vi "Update Stim Pattern.vi"(0 "Stim Pattern In":T1[][](array[typedef])=[[enum."Full", enum."Half", enum."Off", enum."Off", enum."Off", enum."Off", enum."Half"], [enum."Full", enum."Off", enum."Off", enum."Off", enum."Off", enum."Half", enum."Half"], [enum."Half", enum."Full", enum."Off", enum."Full", enum."Off", enum."Off", enum."Full"], [enum."Half", enum."Off", enum."Off", enum."Half", enum."Full", enum."Full", enum."Full"], [enum."Off", enum."Full", enum."Half", enum."Half", enum."Off", enum."Off", enum."Off"]]) -> (1 "Stim Pattern Out":T1[][](array[typedef])=[[enum."Full", enum."Half", enum."Off", enum."Off", enum."Off", enum."Off", enum."Half"], [enum."Full", enum."Off", enum."Off", enum."Off", enum."Off", enum."Half", enum."Half"], [enum."Half", enum."Full", enum."Off", enum."Full", enum."Off", enum."Off", enum."Full"], [enum."Half", enum."Off", enum."Off", enum."Half", enum."Full", enum."Full", enum."Full"], [enum."Off", enum."Full", enum."Half", enum."Half", enum."Off", enum."Off", enum."Off"]], 2 "Pretty Colors Out":u32[][](array[colorbox]))   [LabVIEW 2019]
uses:
  Gait Phase Names.ctl
  Stim off-half-ful.ctl
  Muscle Group Labels.ctl
panel:
  out "Pretty Colors Display":T4={"Muscle Group Labels"=["Muscle Groups", "Gluteals", "Hamstrings", "Quadriceps", "Tibialis Anterior", "Triceps Surae"], "Cluster"={"Gait Phases  "=["LR", "MSt", "TSt", "PSw", "ISw", "MSw", "TSw"], "Pretty Colors"=[]}}
  in  "Stim Pattern Control":T5={"_"={"Array 3"=["Muscle Groups"], "Array 2"=["Gluteals", "Hamstrings", "Quadriceps", "Tibialis Anterior", "Triceps Surae"]}, "Stimulation Pattern"={"Gait Phases  "=["LR", "MSt", "TSt", "PSw", "ISw", "MSw", "TSw"], "Values"=[[enum."Full", enum."Half", enum."Off", enum."Off", enum."Off", enum."Off", enum."Half"], [enum."Full", enum."Off", enum."Off", enum."Off", enum."Off", enum."Half", enum."Half"], [enum."Half", enum."Full", enum."Off", enum."Full", enum."Off", enum."Off", enum."Full"], [enum."Half", enum."Off", enum."Off", enum."Half", enum."Full", enum."Full", enum."Full"], [enum."Off", enum."Full", enum."Half", enum."Half", enum."Off", enum."Off", enum."Off"]]}}
  in  "F'n Done":bool
  # "Edit Here"
  # "Pretty Colors"
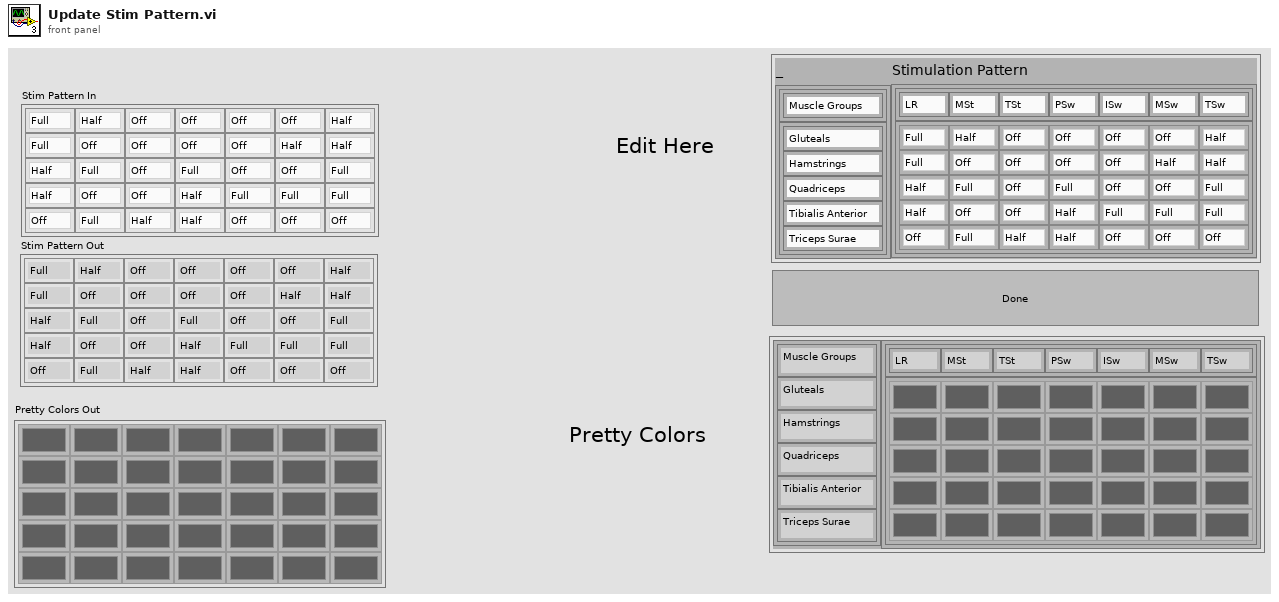
[diagram p1: front panel]
types:
  T1 = typedef "Stim off-half-ful.ctl" = enum16{"Off", "Half", "Full"}
  T2 = typedef "Muscle Group Labels.ctl" = string[]
  T3 = typedef "Gait Phase Names.ctl" = string[]
  T4 = cluster{"Muscle Group Labels":T2, "Cluster":cluster{"Gait Phases  ":T3, "Pretty Colors":u32[][]}}
  T5 = cluster{"_":cluster{"Array 3":string[], "Array 2":string[]}, "Stimulation Pattern":cluster{"Gait Phases  ":T3, "Values":T1[][]}}
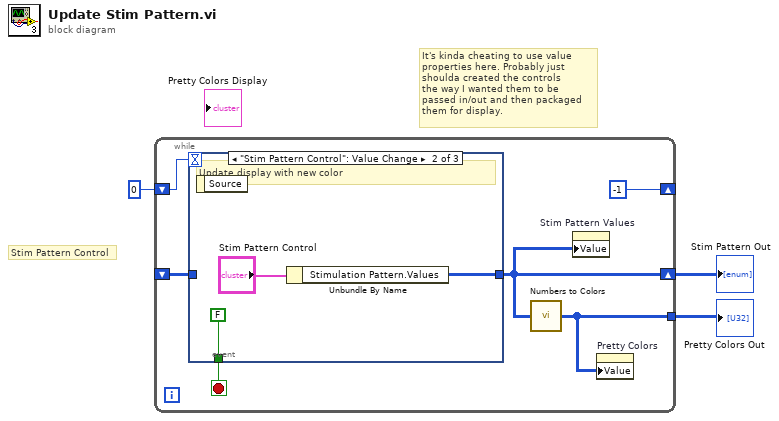
[diagram p0: block diagram]
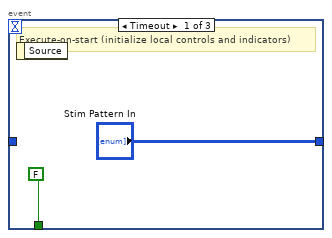
[diagram p2: hidden frame]
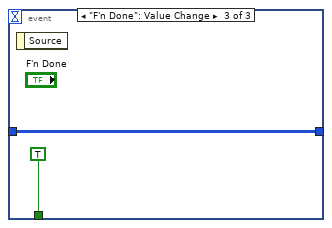
[diagram p3: hidden frame]
diagram:
  # "It's kinda cheating to use value\nproperties here. Probably just\nshoulda created the controls\nthe way I wanted them to be\npassed in/out and then packaged\nthem for display."
  # "Stim Pattern Control"
  n1 = while {
    shift-right: [-1] -> _
    shift-left: 0 -> [w8]
    shift-right: [w6] -> w2
    shift-left: _ -> [w5]
    tunnel: [w4] -> w1
    stop <- w9 stop-if-true
    n2 = event shown="[1] \"Stim Pattern Control\": Value Change" {
      selector: _ -> [_ _ _]
      dyn-events: _ -> [_ _ _]
      timeout: w8 -> [_ _ _]
      tunnel: [FALSE FALSE TRUE] -> w9
      tunnel: ["Stim Pattern In" w12 w15] -> w6
      tunnel: w5 -> [_ _ w15]
      event Timeout {
        # "Execute-on-start (initialize local controls and indicators)"
        n3 = event-data() -> ()  [unwired: 1 in, 1 out]
      }
      event "Stim Pattern Control": Value Change {
        # "Update display with new color"
        n4 = event-data() -> ()  [unwired: 1 in, 1 out]
        n5 = Unbundle By Name("Stim Pattern Control") -> ("Stimulation Pattern.Values"=w12:T1[][])
      }
      event "F'n Done": Value Change {
        n6 = event-data() -> ()  [unwired: 1 in, 1 out]
      }
    }
    n7 = call "Numbers to Colors.vi"("Left Stim Pattern Values"=w6) -> ("Stim Pattern Array"=w4:u32[][])
    n8 = property on="Stim Pattern Values" class="Arr (strict)"("Value"=w6) -> ()  [unwired: 2 in, 2 out]
    n9 = property on="Pretty Colors" class="Arr (strict)"("Value"=w4) -> ()  [unwired: 2 in, 2 out]
  }
  "Stim Pattern Out" <- w2
  "Pretty Colors Out" <- w1
